vi "E710_WaveGenerator_Sample_Program.vi"(0 "System no.":i32=1 min=1 max=4 step=1, 2 "Affected axis":string, 3 "Choice":bool[](array[boolean])=[FALSE, FALSE, FALSE, FALSE, FALSE, FALSE, FALSE, FALSE, FALSE, FALSE, FALSE, FALSE, FALSE, FALSE, FALSE, FALSE, FALSE, FALSE, FALSE, FALSE, FALSE, FALSE, FALSE, FALSE, FALSE, FALSE, FALSE, FALSE, FALSE, FALSE, FALSE, FALSE], 4 "DDL":bool, 5 "error in":errorcluster, 6 "Xo (Start)":i32, 7 "SIN_P Parameters":cluster{"C":dbl, "A":dbl, "O":dbl}={"C"=200.0, "A"=50.0, "O"=0.0} {"O" format="%.6f"; "A" format="%.6f"; "C" format="%.6f"}, 8 "N (Length)":i32=500 min=0 max=1000 step=1, 9 "Append? (&)":bool, 10 "Xo (Start)":i32, 11 "RAMP Parameters":cluster{"C":dbl, "J":dbl, "A":dbl, "O":dbl}={"C"=200.0, "J"=0.0, "A"=20.0, "O"=0.0} {"O" format="%.6f"; "A" format="%.6f"; "J" format="%.6f"; "C" format="%.6f"}, 12 "N (Length)":i32=500 min=0 max=1000 step=1, 13 "Append? (&)":bool) -> (19 "Error out":errorcluster)   [LabVIEW 2010]
doc: "This VI demonstrates how to use the wave generator command VI's of the E-710. It first moves the affected axis to a start position of zero. Then it runs in a loop, giving the user the options to write sine wave curve segments or ramps into the E-710 wave buffer. Wave storage data points are limited to 1000 points to keep transfer times low. The segment length of one waveform - which normally defines the frequency - is predefined as 500 points in this example. Depending on the value of Append? (&), either the old buffer data is overwritten or the new wave will be appended to memory. Please take into account that you can append at most two waveforms since buffer size is limited to 1000 points as mentioned above. \n\nAdjust the following controls to modify the shape of the waveforms.\nN (Length): Waveform (i.e. the points to be modified) goes from 0 to Length. Datapoints from Length to 500 are filled with zeros.\nXo (Start): Position where the first point of the waveform is located. \nC: Center point of the wave. If C = Length/2 then the wave is symmetrical.\nA: Amplitude of the waveform. F(x) = A*sin(x) + O\nO: Offset of the waveform. F(x) = A*sin(x) + O\nJ: Jerk. Means curvature in the transition to or from standstill.\n\nYou have to stop generator output prior to restarting it with a different parameter set. Otherwise you get a Hidden error. The Start Gen. and Stop Gen. buttons will enable or disable the wave generator output by sending \"WGO 0\" or \"WGO 1\" for the affected axis. The red Stop button stops the wave generator output on the specified axis and finishes the loop. \n\nPlease respect the delays that occur while the controller is processing your commands. This is indicated by the Writing... indicator. \n\nIn case of an error a button \"Clear Error\" will appear and the control buttons above will be disabled. Pressing this button will clear the error status and enable the control buttons again.\n\nWith DDL ON you can achieve significantly better position accuracy. Compare the target (green), response (white) and error (red) signals on the graph. Since this is a very sensitive mechanism we recommend starting with low amplitudes and adjusting the parameters with caution. The DDL button works only if the controller supports DDL. Contact PI for information on activation of DDL support.\nRun E710_Configuration_Setup prior to running this VI. \n\nValid for: E-710"
panel:
  out "DDL":bool
  in  "Clear Error":bool
  out "Busy?":bool
  out "Hidden error":bool
  in  "Stop wave generator \noutput":bool
  # "E-710 wave generator sample program"
  # "This VI demonstrates how to use the wave generator command VIs of the E-710. It first moves the affected axis to a start position of zero. Then it runs in a \nloop, giving the user the options to write sine wave curve segments or ramps into the E-710 wave buffer. Wave storage data points are limited to 1000 points\nto keep transfer times low. The segment length of one waveform is predefined as 500 points in this example. Depending on the value of Append? (&), either\nthe old buffer data is overwritten or the new wave will be appended to memory. You have to stop generator output prior to restarting it with a different\nparameter set. The Start Gen. and Stop Gen. buttons will enable or disable the wave generator output by sending \"WGO 0\" or \"WGO 1\" for the affected axis. \nIf DDL is enabled \"WGO 65\" will be sent respectively. The red Stop button stops the wave generator output on the specified axis and finishes the loop. \nPlease respect the delays that occur while the controller is processing your commands. This is indicated by the \"Busy?\" indicator. See manual for further details. \nRun E710_Configuration_Setup prior to running this VI."
  # "Sine Parameters:"
  # "Ramp Parameters:"
  # "Write Sine"
  # "Write Ramp"
  # "Start Gen"
  # "DDL state"
  # "Stop Gen"
  # "Stop\nwave\ngenerator\noutput"
  # "Read Buffer"
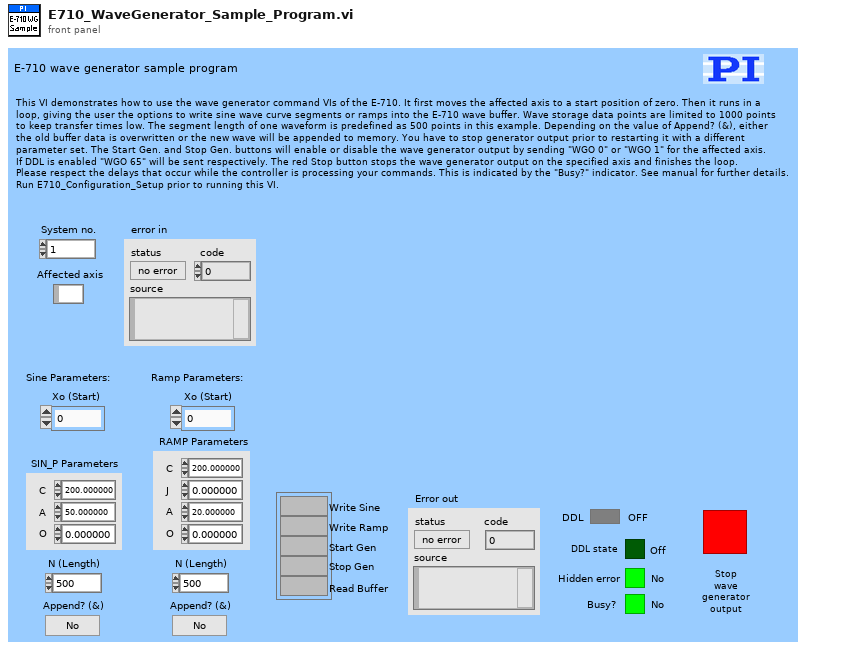
[diagram p1: front panel]
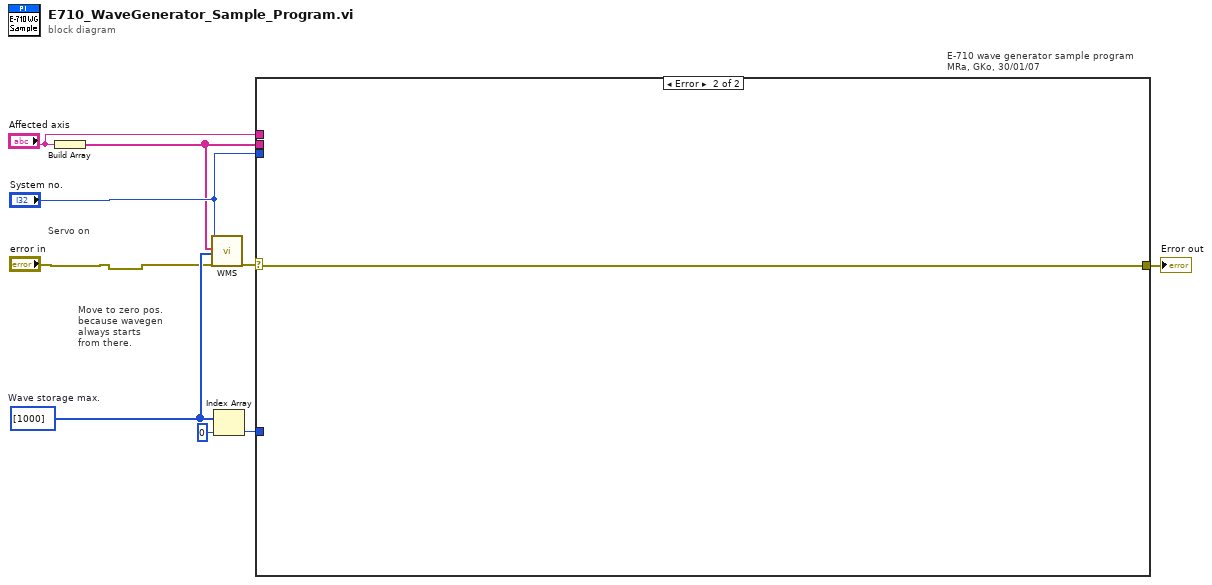
[diagram p0: block diagram]
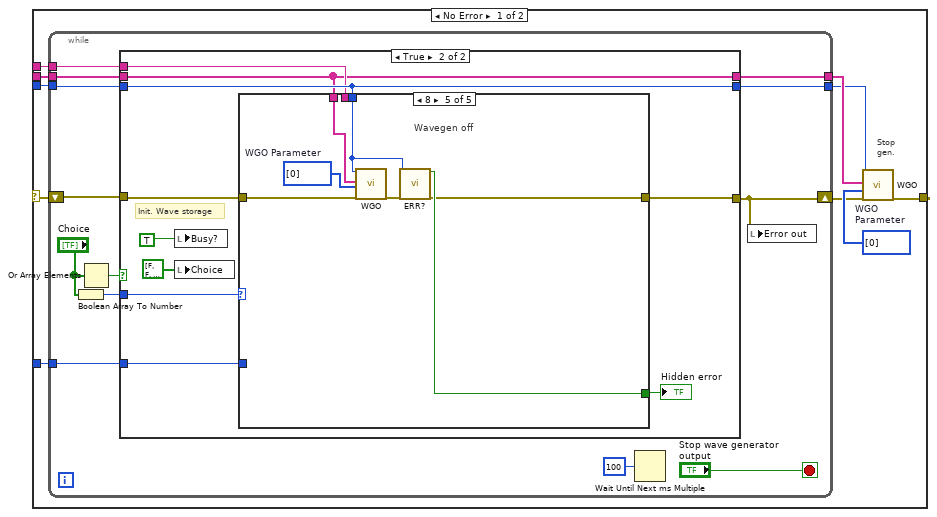
[diagram p2: hidden frame]
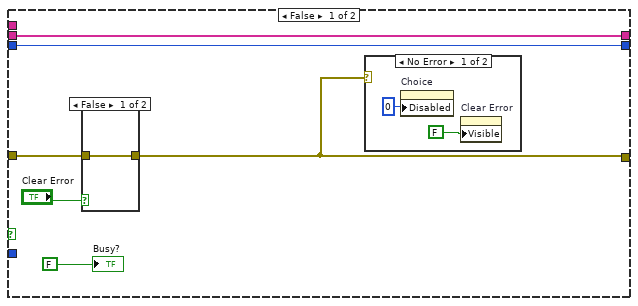
[diagram p3: hidden frame]
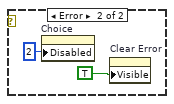
[diagram p4: hidden frame]
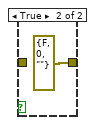
[diagram p5: hidden frame]
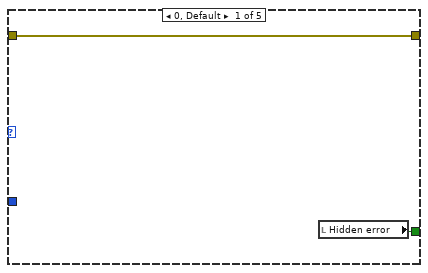
[diagram p6: hidden frame]
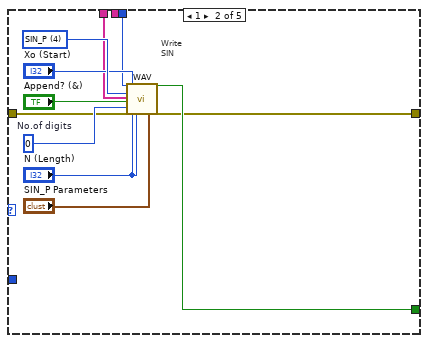
[diagram p7: hidden frame]
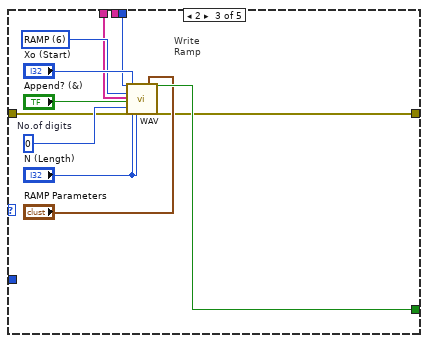
[diagram p8: hidden frame]
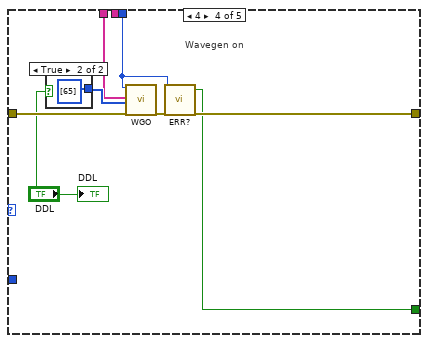
[diagram p9: hidden frame]
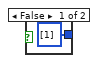
[diagram p10: hidden frame]
diagram:
  w4 = i32[] [1000]  # Wave storage max.
  # "Servo on"
  # "Move to zero pos.\nbecause wavegen\nalways starts \nfrom there."
  # "E-710 wave generator sample program\nMRa, GKo, 30/01/07"
  n1 = Build Array("Affected axis") -> (w7:string[])
  n2 = call "WMS.vi"("System no."="System no.", "Axes to set"=w7, "Wave storage max."=w4, "error in"="error in") -> ("error out"=w6:errorcluster)  [unwired: 14 in, 1 out]
  n3 = Index Array(array=w4, index=0 ("Index")) -> (element=w5:i32)
  n4 = case shown="Error" w6 {
    selector: w6 -> [w12 w96]
    tunnel: w7 -> [w19 _]
    tunnel: "System no." -> [w18 _]
    tunnel: [w17 w96] -> w9
    tunnel: w5 -> [w11 _]
    tunnel: "Affected axis" -> [w10 _]
    frame No Error {
      w16 = i32[] [0]  # WGO  Parameter
      # "Stop\ngen."
      n5 = while {
        tunnel: w19 -> [w27]
        tunnel: w18 -> [w25]
        tunnel: [w26] -> w15
        tunnel: [w24] -> w14
        shift-right: [w22] -> w13
        shift-left: w12 -> [w23]
        tunnel: w11 -> [w21]
        tunnel: w10 -> [w20]
        stop <- "Stop wave generator \noutput" stop-if-true
        n6 = Boolean Array To Number(Boolean array="Choice") -> (number=w30:u32)
        n7 = Or Array Elements(Boolean array="Choice") -> (logical OR=w29:bool)
        n8 = case shown="True" w29 {
          tunnel: [w33 w50] -> w22
          tunnel: w30 -> [_ w52]
          tunnel: w25 -> [w37 w49]
          tunnel: w27 -> [w36 w45]
          tunnel: [w36 w45] -> w26
          tunnel: [w37 w49] -> w24
          tunnel: w23 -> [w35 w51]
          tunnel: w21 -> [_ w47]
          tunnel: w20 -> [_ w46]
          frame False {
            n9 = case shown="False" "Clear Error" {
              tunnel: w35 -> [w43 _]
              tunnel: [w43 errorcluster {"status"=FALSE, "code"=0, "source"=""} ("error IO")] -> w33
              frame False {
              }
              frame True {
              }
            }
            n10 = case shown="No Error" w33 {
              frame No Error {
                n11 = property on="Choice" class="Arr (strict)"("Disabled"=u8 0) -> ()  [unwired: 2 in, 2 out]
                n12 = property on="Clear Error" class="Bool"("Visible"=FALSE) -> ()  [unwired: 2 in, 2 out]
              }
              frame Error {
                n13 = property on="Choice" class="Arr (strict)"("Disabled"=u8 2) -> ()  [unwired: 2 in, 2 out]
                n14 = property on="Clear Error" class="Bool"("Visible"=TRUE) -> ()  [unwired: 2 in, 2 out]
              }
            }
            "Busy?" <- FALSE
          }
          frame True {
            # "Init. Wave storage"
            n15 = local write "Busy?"(TRUE) -> ()
            n16 = local write "Choice"(bool[] [FALSE, FALSE, FALSE, FALSE, FALSE, FALSE, FALSE, FALSE, FALSE, FALSE, FALSE, FALSE, FALSE, FALSE, FALSE, FALSE, FALSE, FALSE, FALSE, FALSE, FALSE, FALSE, FALSE, FALSE, FALSE, FALSE, FALSE, FALSE, FALSE, FALSE, FALSE, FALSE] ("Choice")) -> ()
            n17 = case shown="8" w52 {
              tunnel: [w56 w62 w74 w82 w93] -> w48
              tunnel: [w55 w61 w72 w84 w91] -> w50
              tunnel: w51 -> [w55 w60 w71 w85 w94]
              tunnel: w46 -> [_ _ _ _ _]
              tunnel: w49 -> [_ w59 w70 w80 w90]
              tunnel: w47 -> [_ _ _ _ _]
              tunnel: w45 -> [_ w58 w69 w79 w89]
              frame 0, Default {
                n18 = local read "Hidden error"() -> (w56:bool)
              }
              frame 1 {
                w64 = i16 0  # No.of digits
                w67 = u16 4 items=["SIN", "POL", "TAN", "PNT", "SIN_P", "LIN", "RAMP"] ("Waveform")
                # "Write\nSIN"
                n19 = call "WAV.vi"("System no."=w59, "Waveform"=w67, "Affected axes"=w58, "Append? (&)"="Append? (&)", "No.of digits"=w64, "error in"=w60, "Xo"="Xo (Start)", "N"="N (Length)", "Segment length"="N (Length)", "SIN_P Parameters"="SIN_P Parameters") -> ("Hidden error"=w62:bool, "error out"=w61:errorcluster)  [unwired: 16 in]
              }
              frame 2 {
                w75 = u16 6 items=["SIN", "POL", "TAN", "PNT", "SIN_P", "LIN", "RAMP"] ("Waveform")
                w77 = i16 0  # No.of digits
                # "Write\nRamp"
                n20 = call "WAV.vi"("System no."=w70, "Waveform"=w75, "Affected axes"=w69, "Append? (&)"="Append? (&)", "No.of digits"=w77, "error in"=w71, "Xo"="Xo (Start)", "N"="N (Length)", "Segment length"="N (Length)", "RAMP Parameters"="RAMP Parameters") -> ("Hidden error"=w74:bool, "error out"=w72:errorcluster)  [unwired: 16 in]
              }
              frame 4 {
                # "Wavegen on"
                n21 = case shown="True" "DDL" {
                  tunnel: [i32[] [1] ("WGO Parameter") i32[] [65] ("WGO Parameter")] -> w86
                  frame False {
                  }
                  frame True {
                  }
                }
                n22 = call "WGO.vi"("System no."=w80, "Affected axes"=w79, "WGO Parameter"=w86, "error in"=w85) -> ("error out"=w83:errorcluster)  [unwired: 14 in, 1 out]
                n23 = call "ERR?.vi"("System no."=w80, "error in"=w83) -> ("Hidden error"=w82:bool, "error out"=w84:errorcluster)  [unwired: 16 in]
                "DDL" <- "DDL"
              }
              frame 8 {
                w95 = i32[] [0]  # WGO Parameter
                # "Wavegen off"
                n24 = call "WGO.vi"("System no."=w90, "Affected axes"=w89, "WGO Parameter"=w95, "error in"=w94) -> ("error out"=w92:errorcluster)  [unwired: 14 in, 1 out]
                n25 = call "ERR?.vi"("System no."=w90, "error in"=w92) -> ("Hidden error"=w93:bool, "error out"=w91:errorcluster)  [unwired: 16 in]
              }
            }
            "Hidden error" <- w48
          }
        }
        n26 = Wait Until Next ms Multiple(millisecond multiple=u32 100) -> ()  [unwired: 1 out]
        n27 = local write "Error out"(w22) -> ()
      }
      n28 = call "WGO.vi"("System no."=w14, "Affected axes"=w15, "WGO Parameter"=w16, "error in"=w13) -> ("error out"=w17:errorcluster)  [unwired: 14 in, 1 out]
    }
    frame Error {
    }
  }
  "Error out" <- w9
